vi "PhotonPoseEstimator_closestToCameraHeightStrategy_calc.vi"(4 "TimeStamp":dbl, 6 "FieldTargetPose":T7={"Translation3d"={"X"=0.0, "Y"=0.0, "Z"=0.0}, "Rotation3d"={"Q_quaternion"={"R"=1.0, "V"=[0.0, 0.0, 0.0]}}} {"Translation3d"."Z" format="%14.3f"; "Translation3d"."Y" format="%14.3f"; "Translation3d"."X" format="%14.3f"}, 7 "RobotToCam":T3={"TRANSLATION3D"={"X"=0.0, "Y"=0.0, "Z"=0.0}, "ROTATION3D"={"Q_quaternion"={"R"=1.0, "V"=[0.0, 0.0, 0.0]}}, "XF"=FALSE} {"TRANSLATION3D"."Z" format="%14.3f"; "TRANSLATION3D"."Y" format="%14.3f"; "TRANSLATION3D"."X" format="%14.3f"}, 8 "Targets":T1[](array[typedef]) {"AltCameraToTarget"."TRANSLATION3D"."Z" format="%14.3f"; "AltCameraToTarget"."TRANSLATION3D"."Y" format="%14.3f"; "AltCameraToTarget"."TRANSLATION3D"."X" format="%14.3f"; "BestCameraToTarget"."TRANSLATION3D"."Z" format="%14.3f"; "BestCameraToTarget"."TRANSLATION3D"."Y" format="%14.3f"; "BestCameraToTarget"."TRANSLATION3D"."X" format="%14.3f"}, 9 "TransformToEvaluate":T3={"TRANSLATION3D"={"X"=0.0, "Y"=0.0, "Z"=0.0}, "ROTATION3D"={"Q_quaternion"={"R"=1.0, "V"=[0.0, 0.0, 0.0]}}, "XF"=FALSE} {"TRANSLATION3D"."Z" format="%14.3f"; "TRANSLATION3D"."Y" format="%14.3f"; "TRANSLATION3D"."X" format="%14.3f"}, 10 "SmallestHeightDiff":dbl, 11 "CurrentBestTrackedTarg":T8={"EstimatedPose"={"Translation3d"={"X"=0.0, "Y"=0.0, "Z"=0.0}, "Rotation3d"={"Q_quaternion"={"R"=1.0, "V"=[0.0, 0.0, 0.0]}}}, "TimeStamp_Seconds"=0.0, "targetsUsed"=[], "Strategy"=enum."LOWEST_AMBIGUITY"} {"targetsUsed"."AltCameraToTarget"."TRANSLATION3D"."Z" format="%14.3f"; "targetsUsed"."AltCameraToTarget"."TRANSLATION3D"."Y" format="%14.3f"; "targetsUsed"."AltCameraToTarget"."TRANSLATION3D"."X" format="%14.3f"; "targetsUsed"."BestCameraToTarget"."TRANSLATION3D"."Z" format="%14.3f"; "targetsUsed"."BestCameraToTarget"."TRANSLATION3D"."Y" format="%14.3f"; "targetsUsed"."BestCameraToTarget"."TRANSLATION3D"."X" format="%14.3f"; "EstimatedPose"."Translation3d"."Z" format="%14.3f"; "EstimatedPose"."Translation3d"."Y" format="%14.3f"; "EstimatedPose"."Translation3d"."X" format="%14.3f"}) -> (1 "Found New Best":bool, 2 "SmallestHieghtDiff":dbl, 3 "PhotonEstimatedRobotPose":T8={"EstimatedPose"={"Translation3d"={"X"=0.0, "Y"=0.0, "Z"=0.0}, "Rotation3d"={"Q_quaternion"={"R"=1.0, "V"=[0.0, 0.0, 0.0]}}}, "TimeStamp_Seconds"=0.0, "targetsUsed"=[], "Strategy"=enum."LOWEST_AMBIGUITY"} {"targetsUsed"."AltCameraToTarget"."TRANSLATION3D"."Z" format="%14.3f"; "targetsUsed"."AltCameraToTarget"."TRANSLATION3D"."Y" format="%14.3f"; "targetsUsed"."AltCameraToTarget"."TRANSLATION3D"."X" format="%14.3f"; "targetsUsed"."BestCameraToTarget"."TRANSLATION3D"."Z" format="%14.3f"; "targetsUsed"."BestCameraToTarget"."TRANSLATION3D"."Y" format="%14.3f"; "targetsUsed"."BestCameraToTarget"."TRANSLATION3D"."X" format="%14.3f"; "EstimatedPose"."Translation3d"."Z" format="%14.3f"; "EstimatedPose"."Translation3d"."Y" format="%14.3f"; "EstimatedPose"."Translation3d"."X" format="%14.3f"})   [LabVIEW 2019, in "PhotonVisionLib.lvlib"]
doc: "This is an internal function. Use Update or Update_Pipeline instead of this function.\n\nDetermine the best target based on the target height closed to the camera height."
uses:
  PhotonVisionLib.lvlib
  <vilib>/Rock Robotics/WPI/ThirdParty/JAS_Junk/TrajLib/Trajectory_Library.lvlib
  Enum/PhotonPoseStrategy_ENUM.ctl
  <vilib>/Rock Robotics/WPI/ThirdParty/JAS_Junk/TrajLib/TypeDef/TRANSLATION3D.ctl
  <vilib>/Rock Robotics/WPI/ThirdParty/JAS_Junk/TrajLib/TypeDef/QUATERNION.ctl
  <vilib>/Rock Robotics/WPI/ThirdParty/JAS_Junk/TrajLib/TypeDef/ROTATION3D.ctl
  <vilib>/Rock Robotics/WPI/ThirdParty/JAS_Junk/TrajLib/TypeDef/TRANSFORM3D.ctl
  <vilib>/Rock Robotics/WPI/ThirdParty/JAS_Junk/TrajLib/TypeDef/POSE3D.ctl
  TypeDef/PhotonEstimatedRobotPoseType.ctl
  TypeDef/TargetCornerType.ctl
  TypeDef/PhotonTrackedTargetType.ctl
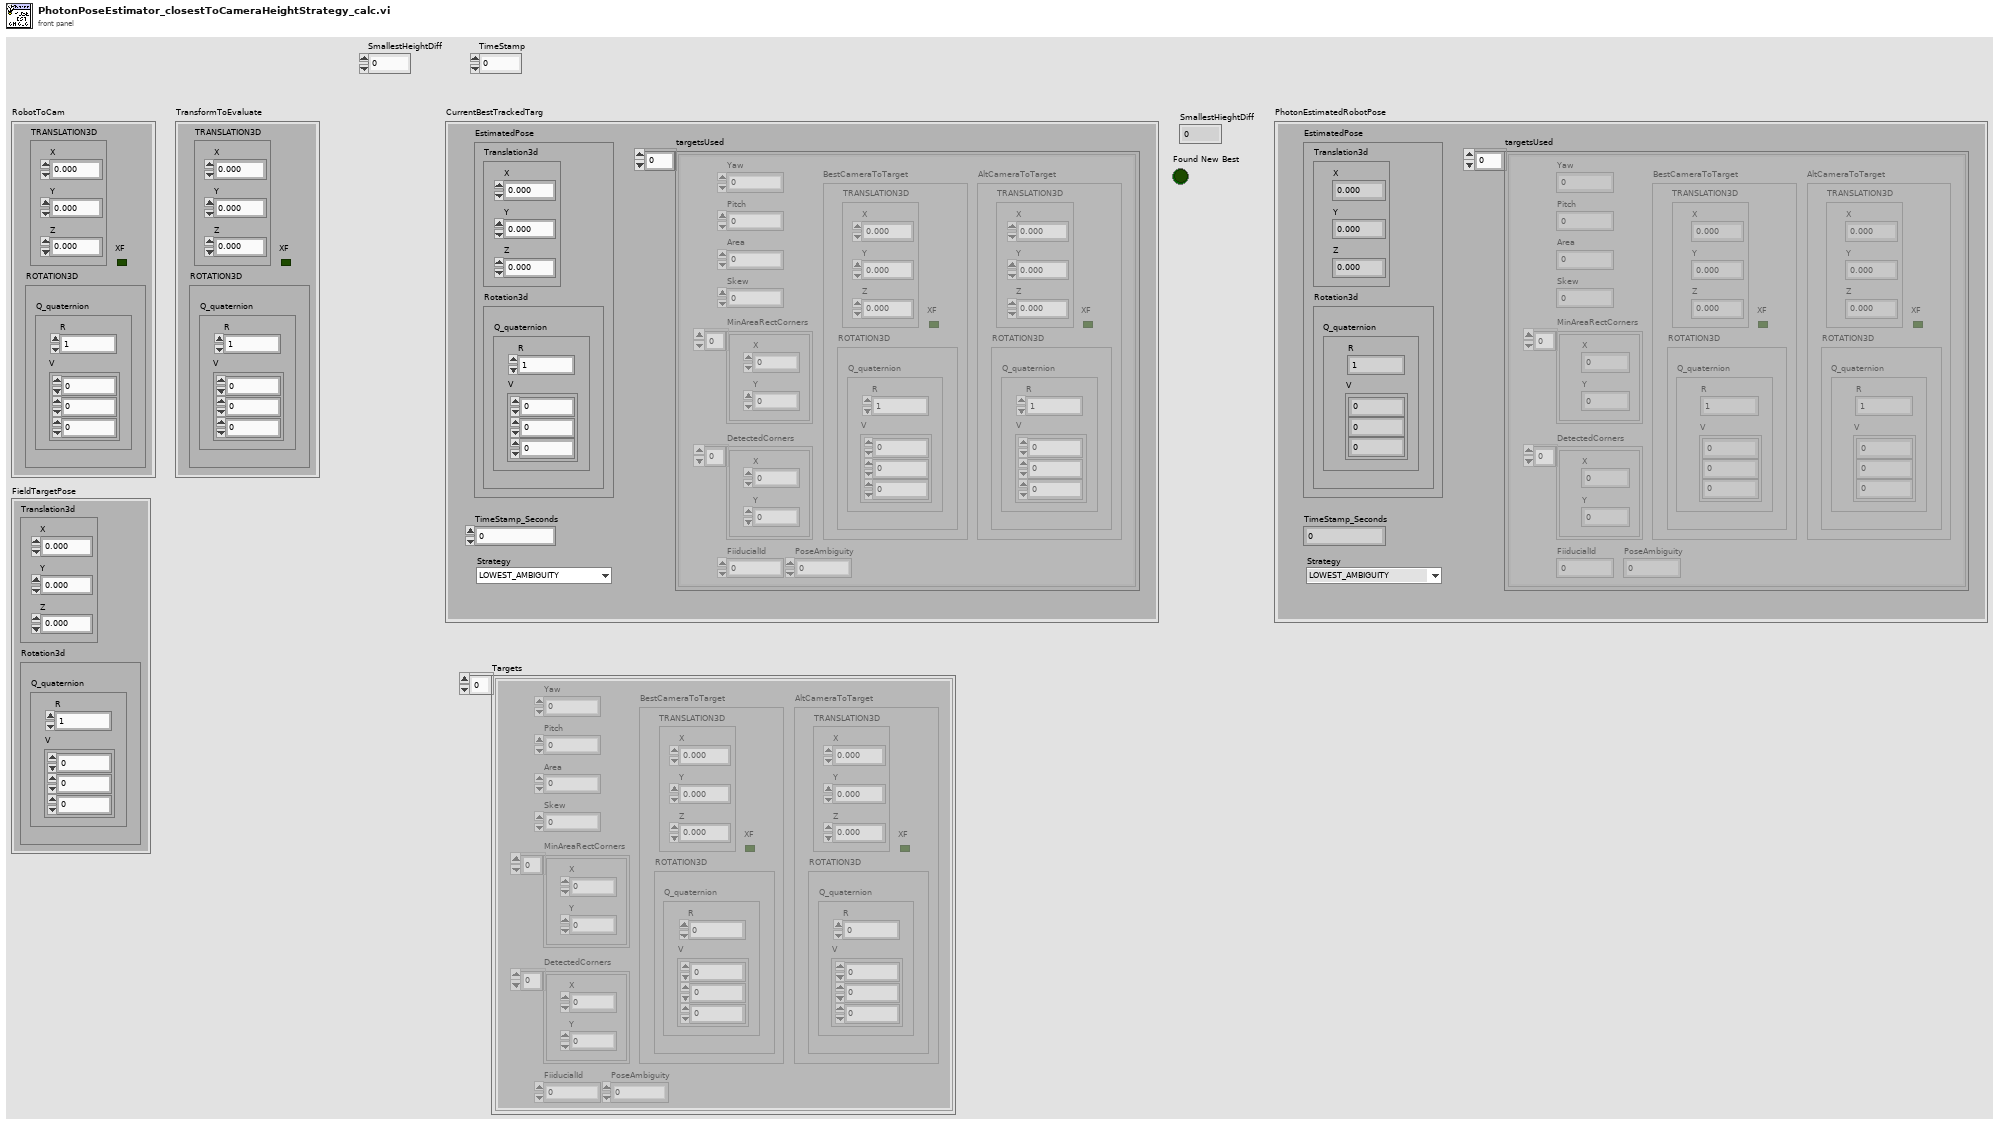
[diagram p1: front panel]
types:
  T1 = typedef "PhotonVisionLib.lvlib/PhotonTrackedTargetType.ctl" = cluster{"Yaw":dbl, "Pitch":dbl, "Area":dbl, "Skew":dbl, "MinAreaRectCorners":T2[], "BestCameraToTarget":T3, "FiiducialId":i32, "AltCameraToTarget":T3, "PoseAmbiguity":dbl, "DetectedCorners":T2[]}
  T2 = typedef "PhotonVisionLib.lvlib/TargetCornerType.ctl" = cluster{"X":dbl, "Y":dbl}
  T3 = typedef "Trajectory_Library.lvlib/TRANSFORM3D.ctl" = cluster{"TRANSLATION3D":T4, "ROTATION3D":T5, "XF":bool}
  T4 = typedef "Trajectory_Library.lvlib/TRANSLATION3D.ctl" = cluster{"X":dbl, "Y":dbl, "Z":dbl}
  T5 = typedef "Trajectory_Library.lvlib/ROTATION3D.ctl" = cluster{"Q_quaternion":T6}
  T6 = typedef "Trajectory_Library.lvlib/QUATERNION.ctl" = cluster{"R":dbl, "V":dbl[]}
  T7 = typedef "Trajectory_Library.lvlib/POSE3D.ctl" = cluster{"Translation3d":T4, "Rotation3d":T5}
  T8 = typedef "PhotonVisionLib.lvlib/PhotonEstimatedRobotPoseType.ctl" = cluster{"EstimatedPose":T7, "TimeStamp_Seconds":dbl, "targetsUsed":T1[], "Strategy":T9}
  T9 = typedef "PhotonVisionLib.lvlib/PhotonPoseStrategy_ENUM.ctl" = enum16{"LOWEST_AMBIGUITY", "CLOSEST_TO_CAMERA_HEIGHT", "CLOSEST_TO_REFERENCE_POSE", "CLOSEST_TO_LAST_POSE", "AVERAGE_BEST_TARGETS", "MULTI_TAG_PNP_ON_COPROCESSOR", "MULTI_TAG_PNP_ON_RIO"}
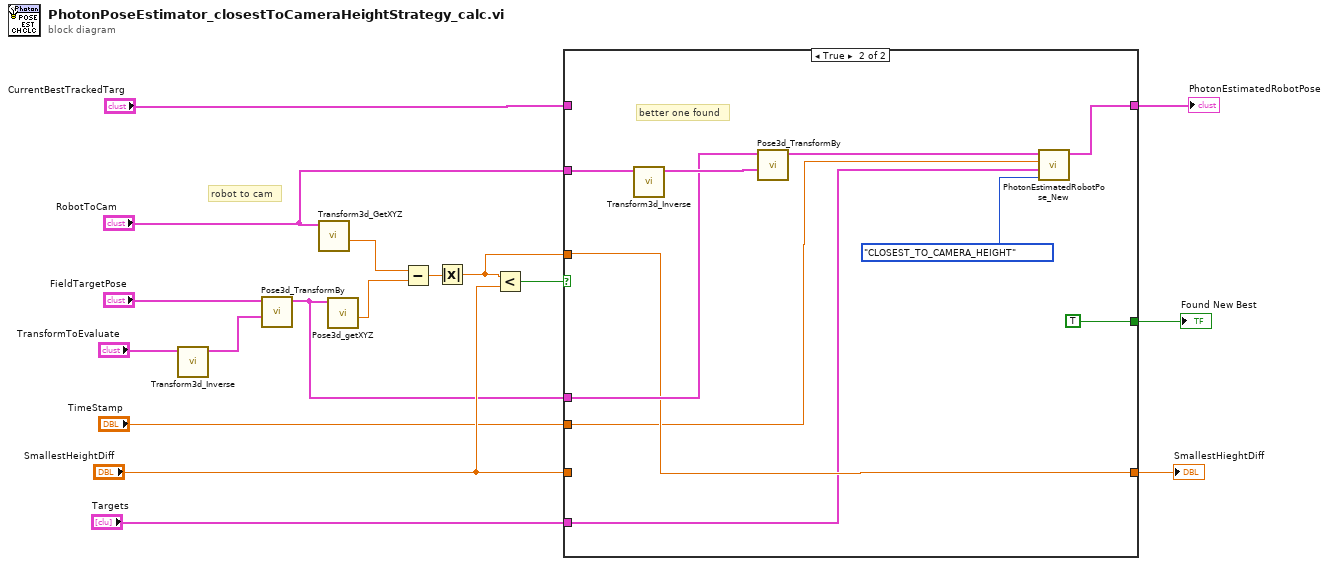
[diagram p0: block diagram]
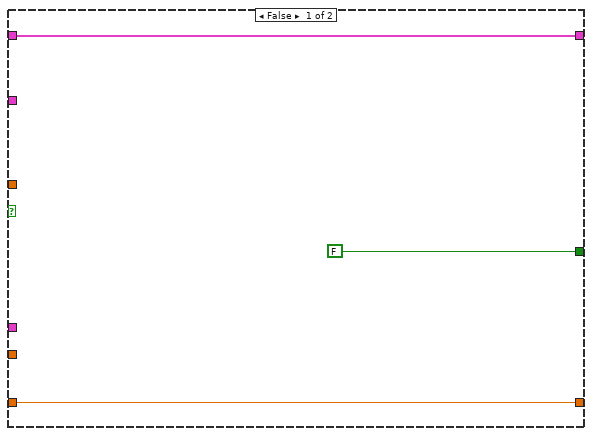
[diagram p2: hidden frame]
diagram:
  # "robot to cam"
  n1 = call <vilib>:"Transform3d_Inverse.vi"("inTransform3d"="TransformToEvaluate") -> ("outTransform3d"=w14:T3)  [unwired: 10 in]
  n2 = call <vilib>:"Pose3d_TransformBy.vi"("other Transform3d"=w14, "in Pose3d"="FieldTargetPose") -> ("out POSE3d"=w4:T7)  [unwired: 9 in]
  n3 = call <vilib>:"Transform3d_GetXYZ.vi"("inTransform3d"="RobotToCam") -> ("Z"=w2:dbl)  [unwired: 8 in, 2 out]
  n4 = call <vilib>:"Pose3d_getXYZ.vi"("in Pose3d"=w4) -> ("Z"=w13:dbl)  [unwired: 8 in, 2 out]
  n5 = Subtract(x=w2, y=w13) -> (x-y=w12:dbl)
  n6 = Absolute Value(x=w12) -> (abs(x)=w7:dbl)
  n7 = Less?(x=w7, y="SmallestHeightDiff") -> (x < y?=w11:bool)
  n8 = case shown="True" w11 {
    tunnel: [FALSE ("Found") TRUE ("Found")] -> w8
    tunnel: "TimeStamp" -> [_ w24]
    tunnel: [w19 w23] -> w17
    tunnel: "CurrentBestTrackedTarg" -> [w19 _]
    tunnel: "SmallestHeightDiff" -> [w18 _]
    tunnel: [w18 w25] -> w9
    tunnel: w7 -> [_ w25]
    tunnel: w4 -> [_ w27]
    tunnel: "RobotToCam" -> [_ w26]
    tunnel: "Targets" -> [_ w21]
    frame False {
    }
    frame True {
      # "better one found"
      n9 = call <vilib>:"Transform3d_Inverse.vi"("inTransform3d"=w26) -> ("outTransform3d"=w29:T3)  [unwired: 10 in]
      n10 = call <vilib>:"Pose3d_TransformBy.vi"("other Transform3d"=w29, "in Pose3d"=w27) -> ("out POSE3d"=w30:T7)  [unwired: 9 in]
      n11 = call "PhotonEstimatedRobotPose_New.vi"("Strategy"=PhotonPoseStrategy_ENUM."CLOSEST_TO_CAMERA_HEIGHT", "targetsUsed"=w21, "TimeStamp_Seconds"=w24, "EstimatedPose"=w30) -> ("PhotonEstimatedRobotPose"=w23:T8)  [unwired: 7 in]
    }
  }
  "Found New Best" <- w8
  "PhotonEstimatedRobotPose" <- w17
  "SmallestHieghtDiff" <- w9
